vi "Convert_RunInfoCluster_2_RunInfoStringList.vi"(2 "error in":errorcluster, 3 "Run Number":string, 4 "Run Data SubPanel Input":T1) -> (0 "error output":errorcluster, 1 "Run Data Output":string)   [LabVIEW 2019]
uses:
  Controls/DataBlockControl.ctl
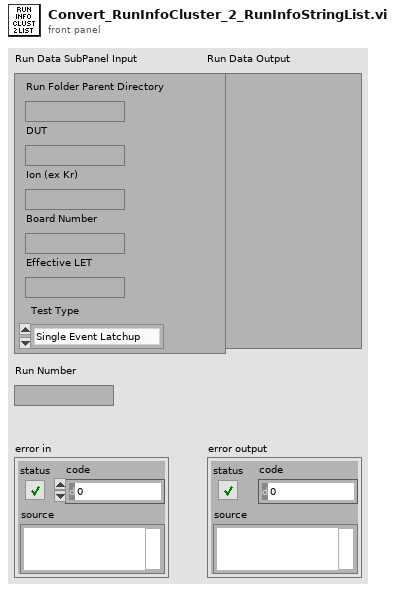
[diagram p1: front panel]
types:
  T1 = typedef "DataBlockControl.ctl" = cluster{"Run Folder Parent Directory":path, "DUT":string, "Ion (ex Kr)":string, "Board Number":string, "Effective LET":string, "Test Type":enum16{"Single Event Latchup", "Single Event Transient", "Single Event Upset"}}
  T2 = enum16{"Single Event Latchup", "Single Event Transient", "Single Event Upset"}
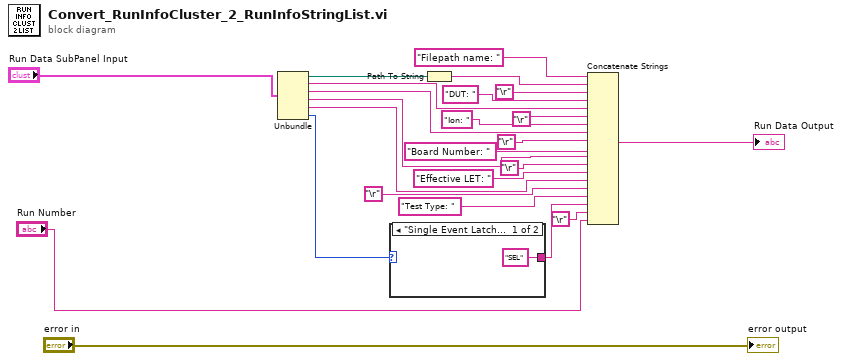
[diagram p0: block diagram]
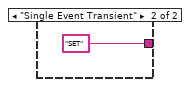
[diagram p2: hidden frame]
diagram:
  n1 = Unbundle("Run Data SubPanel Input") -> ("Run Folder Parent Directory"=w5:path, "DUT"=w10:string, "Ion (ex Kr)"=w13:string, "Board Number"=w16:string, "Effective LET"=w19:string, "Test Type"=w21:T2)
  n2 = case shown="\"Single Event Latchup\", Default" w21 {
    tunnel: ["SEL" "SET"] -> w23
    frame "Single Event Latchup", Default {
    }
    frame "Single Event Transient" {
    }
  }
  n3 = Path To String(path=w5) -> (string=w7:string)
  n4 = Concatenate Strings("Filepath name: " ("string"), w7, "\r", "DUT: " ("string"), w10, "\r", "Ion: " ("string"), w13, "\r", "Board Number: " ("string"), w16, "\r", "Effective LET: " ("string"), w19, "\r", "Test Type: " ("string"), w23, "\r", "Run Number") -> (→"Run Data Output":string)
  "error output" <- "error in"
